vi "DAC Run.vi"(8 "error in":errorcluster, 11 "DAC Vacum Valve in":refnum<class "DAC Vacum Valve.lvclass">) -> (0 "error out":errorcluster, 3 "DAC Vacum Valve out":refnum<class "DAC Vacum Valve.lvclass">)   [LabVIEW 2019, in "DAC.lvlib" / "DAC Vacum Valve.lvclass"]
uses:
  DAC Vacum Valve.lvclass
  C:/Users/krio/Documents/LV_Projects/test-stand/App/DAC/DAC.lvclass
  DAC.lvclass/DAC.ctl
  Results/Results Method.ctl
  DAC Vacum Valve.lvclass/DAC Vacum Valve.ctl
  <vilib>/DAQmx/miscellaneous.llb/DAQmx Fill In Error Info.vi
  DAC.lvclass
  Results/Results.lvlib
  Results/HTS Results/HTS Results.lvclass
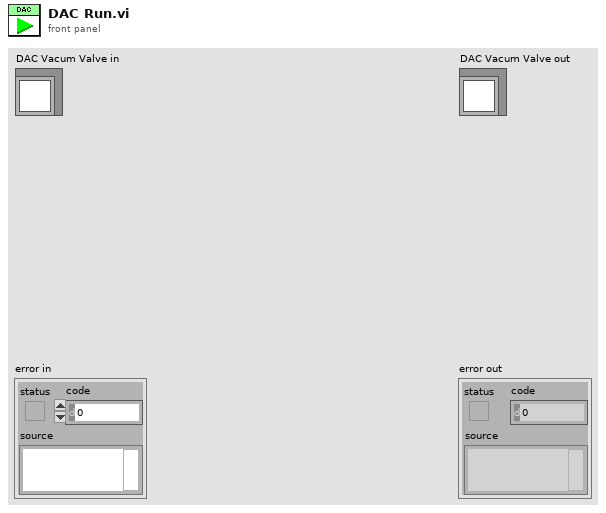
[diagram p1: front panel]
types:
  T1 = typedef "Results.lvlib/Results Method.ctl" = enum16{"Get", "Set"}
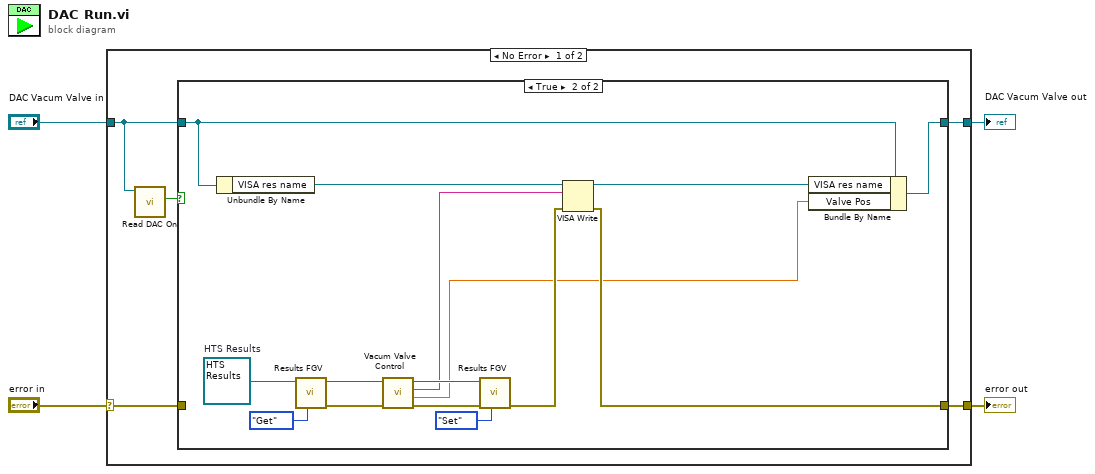
[diagram p0: block diagram]
diagram:
  n1 = case shown="No Error" "error in" {
    selector: "error in" -> [w7 w28]
    tunnel: [w6 w28] -> w2
    tunnel: [w8 w27] -> w1
    tunnel: "DAC Vacum Valve in" -> [w5 w27]
    frame No Error {
      n2 = call "Read DAC On.vi"("DAC in"=w5) -> ("DAC On"=w9:bool)  [unwired: 8 in, 2 out]
      n3 = case shown="True" w9 {
        tunnel: w5 -> [w11 w26]
        tunnel: [w11 w24] -> w8
        tunnel: w7 -> [w10 _]
        tunnel: [w10 w20] -> w6
        frame False {
        }
        frame True {
          w23 = refnum<class "HTS Results.lvclass"> refnum  # HTS Results
          n4 = Unbundle By Name(w26) -> ("VISA res name"=w22:refnum<visa-resource-name>)
          n5 = call-dynamic "Results FGV.vi"("Method"=Results_Method."Get", "HTS Results in"=w23) -> ("error out"=w16:errorcluster, "HTS Results out"=w19:refnum<class "HTS Results.lvclass">)  [unwired: 8 in]
          n6 = call "Vacum Valve Control.vi"("error in"=w16, "HTS Results in"=w19) -> ("error out"=w15:errorcluster, "Valve Pos"=w12:dbl, "Vavum Valve CMD"=w14:string, "HTS Results out"=w17:refnum<class "HTS Results.lvclass">)  [unwired: 6 in]
          n7 = call-dynamic "Results FGV.vi"("Method"=Results_Method."Set", "error in"=w15, "HTS Results in"=w17) -> ("error out"=w13:errorcluster)  [unwired: 7 in, 1 out]
          n8 = VISA Write(VISA resource name=w22, write buffer=w14, error in (no error)=w13) -> (VISA resource name out=w21:refnum<visa-resource-name>, error out=w20:errorcluster)  [unwired: 1 out]
          n9 = Bundle By Name(cluster=w26, "VISA res name"=w21, "Valve Pos"=w12) -> (w24:refnum<class "DAC Vacum Valve.lvclass">)
        }
      }
    }
    frame Error {
    }
  }
  "error out" <- w2
  "DAC Vacum Valve out" <- w1
